vi "server_采集温度风扇.vi"(8 "error in (no error)":errorcluster) -> (0 "error out":errorcluster)   [LabVIEW 2015]
uses:
  Global/SeverGlobal.vi
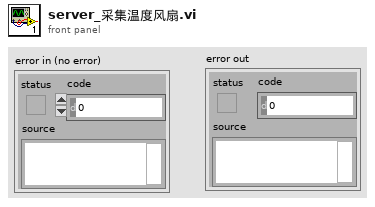
[diagram p1: front panel]
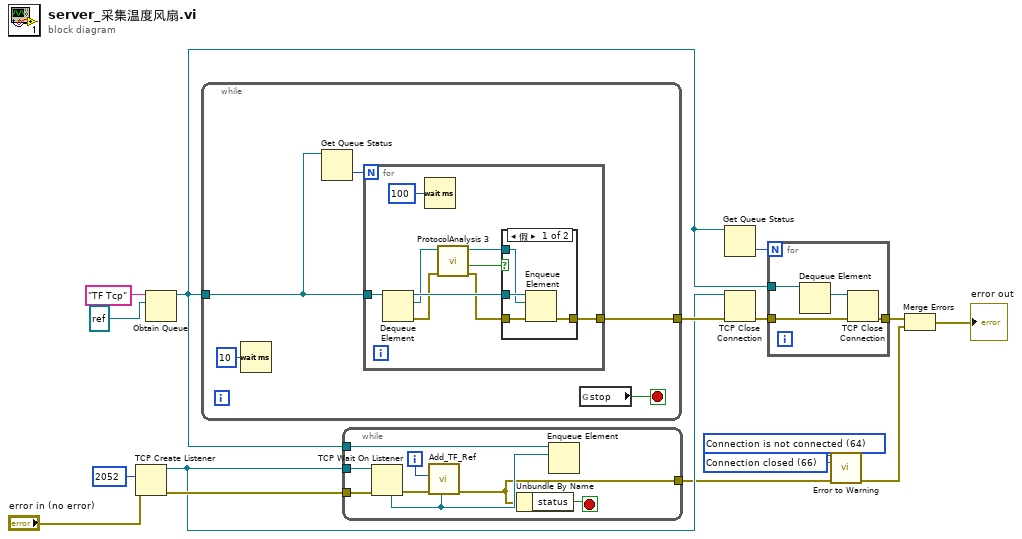
[diagram p0: block diagram]
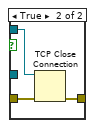
[diagram p2: hidden frame]
diagram:
  w13 = 66 items=["No Error", "Argument Error", "Memory Full", "Out of Zone", "End of File", "File Already Open", "Generic File IO Error", "File Not Found", "File Permission Error", "Disk Full", "Duplicate Path", "Too Many Files Open", "Not Enabled", "Resource File Not Found", "Cannot Add Resource", "Resource Not Found", "Image Not Found", "Image Memory Error", "Pen Does Not Exist", "Config Bad Type", "Config Token Not Found", "Config Parse Error", "Config Memory Error", "Bad External Code Format", "Bad External Code Offset", "External Code Not Present", "Null Window", "Destroy Window Mixup", "Null Menu", "Print Aborted", "Bad Print Record", "Print Driver Error", "Windows Error During Print", "Memory Error During Print", "Print Dialog Error", "Generic Print Error", "Invalid Device Refnum", "Device Not Found", "Device Parameter Error", "Device Unit Error", "Can't Open Device", "Device Call Aborted", "Generic Error", "Cancelled By User", "Object ID Too Low", "Object ID Too High", "Object Not In Heap", "Unknown Heap", "Bad DefProc ID", "DefProc Not In Table", "Message Out Of Range", "Null Method", "Unknown Message", "Manager Call Not Supported", "Bad address", "Connection In progress", "Connection timed out", "Connection is already in progress", "Network attribute not supported", "Network error", "Address in use", "System out of memory", "Connection aborted", "Connection refused", "Connection is not connected", "Connection is already connected", "Connection closed", "Initialize error (interapplication manager)", "Bad occurrence", "Wait on unbound occurrence handler", "Occurrence queue overflow", "Bad path", "Semaphore not signaled", "Unrecognized type (interapplication manager)"] ("2nd Error to Convert")
  w14 = 64 items=["No Error", "Argument Error", "Memory Full", "Out of Zone", "End of File", "File Already Open", "Generic File IO Error", "File Not Found", "File Permission Error", "Disk Full", "Duplicate Path", "Too Many Files Open", "Not Enabled", "Resource File Not Found", "Cannot Add Resource", "Resource Not Found", "Image Not Found", "Image Memory Error", "Pen Does Not Exist", "Config Bad Type", "Config Token Not Found", "Config Parse Error", "Config Memory Error", "Bad External Code Format", "Bad External Code Offset", "External Code Not Present", "Null Window", "Destroy Window Mixup", "Null Menu", "Print Aborted", "Bad Print Record", "Print Driver Error", "Windows Error During Print", "Memory Error During Print", "Print Dialog Error", "Generic Print Error", "Invalid Device Refnum", "Device Not Found", "Device Parameter Error", "Device Unit Error", "Can't Open Device", "Device Call Aborted", "Generic Error", "Cancelled By User", "Object ID Too Low", "Object ID Too High", "Object Not In Heap", "Unknown Heap", "Bad DefProc ID", "DefProc Not In Table", "Message Out Of Range", "Null Method", "Unknown Message", "Manager Call Not Supported", "Bad address", "Connection In progress", "Connection timed out", "Connection is already in progress", "Network attribute not supported", "Network error", "Address in use", "System out of memory", "Connection aborted", "Connection refused", "Connection is not connected", "Connection is already connected", "Connection closed", "Initialize error (interapplication manager)", "Bad occurrence", "Wait on unbound occurrence handler", "Occurrence queue overflow", "Bad path", "Semaphore not signaled", "Unrecognized type (interapplication manager)"] ("1st Error to Convert")
  n1 = TCP Create Listener(8:"error in (no error)", 10:u32 2052 ("端口")) -> (0:w12:errorcluster, 3:w11:refnum<k5>)  [unwired: 3 in, 1 out]
  n2 = Obtain Queue(name (unnamed)="TF Tcp", element data type=refnum<k5> refnum ("listener ID out")) -> (queue out=w2:refnum<queue>)  [unwired: 3 in, 2 out]
  n3 = while {
    tunnel: [w21] -> w15
    tunnel: w2 -> [w20]
    stop <- w18 stop-if-true
    n4 = Wait (ms)(milliseconds to wait=u32 10 ("等待时间（毫秒）")) -> ()  [unwired: 1 out]
    n5 = Get Queue Status(queue=w20) -> (# elements in queue=w17:i32)  [unwired: 2 in, 7 out]
    n6 = for {
      N: w17 -> [_]
      tunnel: [w28] -> w21
      tunnel: w20 -> [w30]
      n7 = Dequeue Element(queue=w30) -> (queue out=w29:refnum<queue>, element=w27:refnum<k5>, error out=w26:errorcluster)  [unwired: 2 in, 1 out]
      n8 = Wait (ms)(milliseconds to wait=u32 100 ("等待时间（毫秒）")) -> ()  [unwired: 1 out]
      n9 = call "ProtocolAnalysis 3.vi"("error in"=w26, "IP"=w27) -> ("error out"=w24:errorcluster, "Disconnected"=w23:bool, "IP 2"=w25:refnum<k5>)  [unwired: 7 in]
      n10 = case shown="假" w23 {
        tunnel: w29 -> [w34 _]
        tunnel: [w33 w35] -> w28
        tunnel: w25 -> [w32 w37]
        tunnel: w24 -> [w31 w36]
        frame False {
          n11 = Enqueue Element(queue=w34, element=w32, error in (no error)=w31) -> (error out=w33:errorcluster)  [unwired: 1 in, 2 out]
        }
        frame True {
          n12 = TCP Close Connection(connection ID=w37, error in (no error)=w36) -> (error out=w35:errorcluster)  [unwired: 1 in, 1 out]
        }
      }
    }
    n13 = global read "SeverGlobal.vi" "stop"() -> (w18:bool)
  }
  n14 = while {
    tunnel: w11 -> [w45]
    tunnel: w12 -> [w44]
    tunnel: [w39] -> w9
    tunnel: w2 -> [w42]
    i -> [w38]
    stop <- w43 stop-if-true
    n15 = TCP Wait On Listener(8:w44, 11:w45) -> (0:w40:errorcluster, 4:w41:refnum<k5>)  [unwired: 2 in, 3 out]
    n16 = call "Add_TF_Ref.vi"("TCP Ref"=w41, "error in"=w40, "index"=w38) -> ("error out"=w39:errorcluster)  [unwired: 8 in]
    n17 = Unbundle By Name(w39) -> ("status"=w43:bool)
    n18 = Enqueue Element(queue=w42, element=w41) -> ()  [unwired: 2 in, 3 out]
  }
  n19 = Get Queue Status(queue=w2) -> (# elements in queue=w4:i32)  [unwired: 2 in, 7 out]
  n20 = TCP Close Connection(connection ID=w11, error in (no error)=w15) -> (error out=w10:errorcluster)  [unwired: 1 in, 1 out]
  n21 = for {
    N: w4 -> [_]
    tunnel: w10 -> [w49]
    tunnel: [w48] -> w8
    tunnel: w2 -> [w47]
    n22 = Dequeue Element(queue=w47) -> (element=w46:refnum<k5>)  [unwired: 2 in, 3 out]
    n23 = TCP Close Connection(connection ID=w46, error in (no error)=w49) -> (error out=w48:errorcluster)  [unwired: 1 in, 1 out]
  }
  n24 = call <vilib>:"Error to Warning.vi"("1st Error to Convert"=w14, "2nd Error to Convert"=w13, "error in"=w9) -> ("warning out"=w7:errorcluster)  [unwired: 12 in]
  n25 = Merge Errors(w8, w7) -> (→"error out":errorcluster)
